vi "Read id.vi"(8 "error in (no error)":errorcluster, 11 "SVG Object in":refnum<class "SVG Object.lvclass">) -> (0 "error out":errorcluster, 2 "id":string, 3 "SVG Object out":refnum<class "SVG Object.lvclass">)   [LabVIEW 2019, in "SVG Object.lvclass"]
uses:
  SVG Object.lvclass
  SVG Object.lvclass/SVG Object.ctl
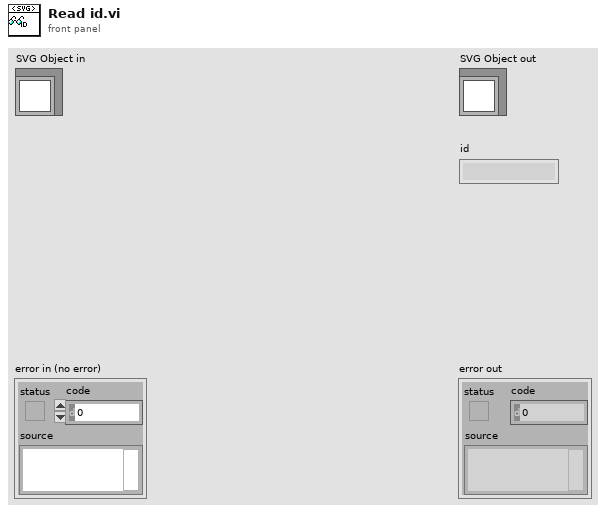
[diagram p1: front panel]
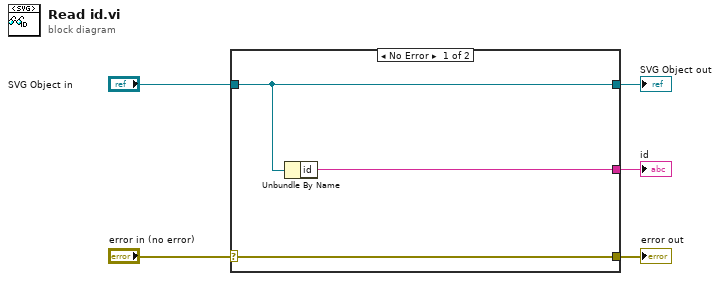
[diagram p0: block diagram]
diagram:
  n1 = case shown="No Error" "error in (no error)" {
    selector: "error in (no error)" -> [w8 w9]
    tunnel: [w8 w9] -> w4
    tunnel: [w7 w10] -> w2
    tunnel: "SVG Object in" -> [w7 w10]
    tunnel: [w6 _] -> w1
    frame No Error {
      n2 = Unbundle By Name(w7) -> ("id"=w6:string)
    }
    frame Error {
    }
  }
  "error out" <- w4
  "SVG Object out" <- w2
  "id" <- w1
